vi "CreateFatalError.vi"(7 "Call Chain? (T)":bool=TRUE, 8 "error in (no error)":errorcluster, 11 "FatalError Text":string) -> (0 "error out":errorcluster)   [LabVIEW 2020, in "NI_XNodeSupport.lvlib"]
uses:
  NI_XNodeSupport.lvlib
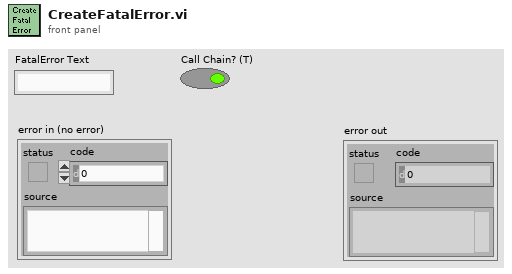
[diagram p1: front panel]
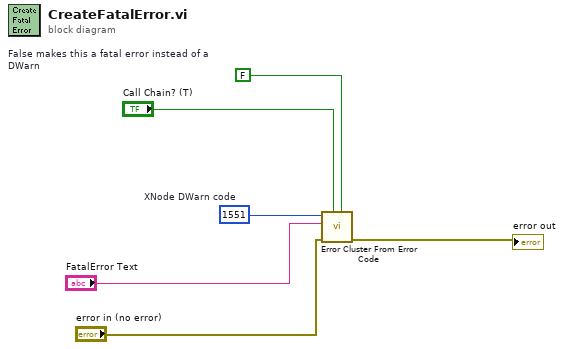
[diagram p0: block diagram]
diagram:
  w5 = FALSE  # False makes this a fatal error instead of a DWarn
  w6 = 1551  # XNode DWarn code
  n1 = call "Error Cluster From Error Code.vi"("is warning? (False)"=w5, "show call chain? (False)"="Call Chain? (T)", "error in (no error)"="error in (no error)", "error message (\"\")"="FatalError Text", "error code (0)"=w6) -> ("error out"=→"error out":errorcluster)  [unwired: 4 in]
